vi "GetColors.vi"(0 "object in":refnum<class "Map.lvclass">, 5 "error in (no error)":errorcluster) -> (14 "object out":refnum<class "Map.lvclass">, 16 "Colors":T1, 19 "error out":errorcluster)   [LabVIEW 2015, in "Map.lvclass"]
uses:
  Map.lvclass
  Map.lvclass/Map.ctl
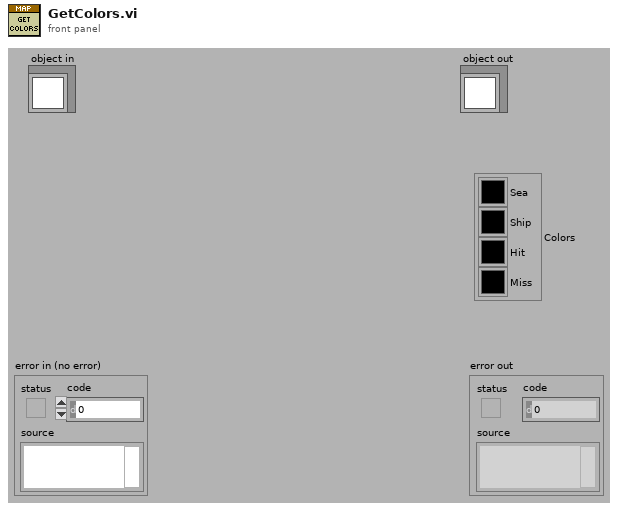
[diagram p1: front panel]
types:
  T1 = cluster{"Sea":u32, "Ship":u32, "Hit":u32, "Miss":u32}
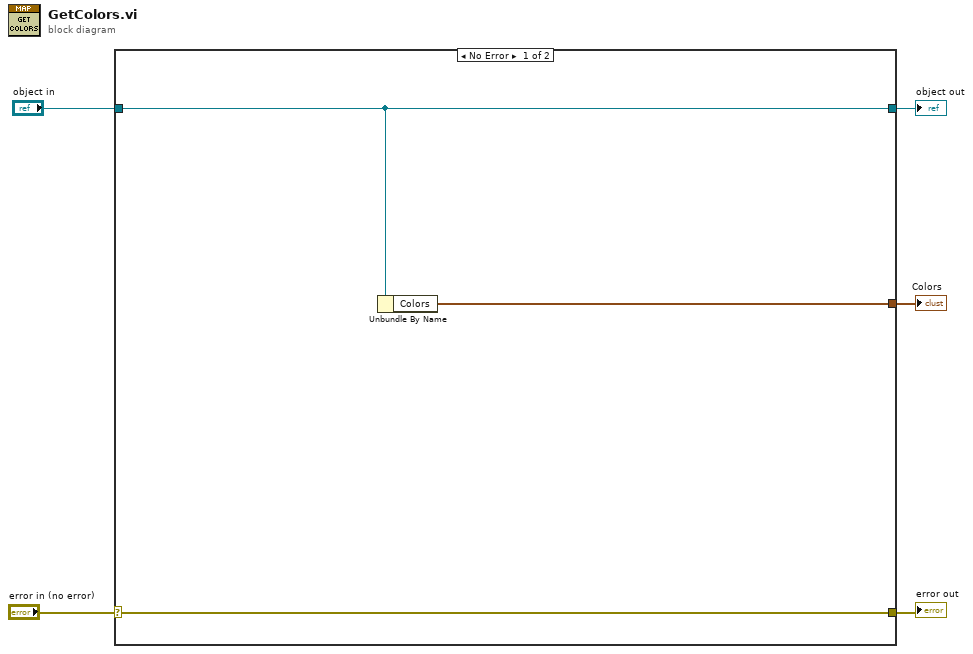
[diagram p0: block diagram]
diagram:
  n1 = case shown="No Error" "error in (no error)" {
    selector: "error in (no error)" -> [w7 w10]
    tunnel: [w7 w10] -> w4
    tunnel: [w6 w9] -> w2
    tunnel: "object in" -> [w6 w9]
    tunnel: [w8 _] -> w1
    frame No Error {
      n2 = Unbundle By Name(w6) -> ("Colors"=w8:T1)
    }
    frame Error {
    }
  }
  "error out" <- w4
  "object out" <- w2
  "Colors" <- w1
